vi "Clear Results.vi"(8 "error in (no error)":errorcluster, 11 "Results Manager in":refnum<class "Results Manager.lvclass">) -> (0 "error out":errorcluster, 3 "Results Manager out":refnum<class "Results Manager.lvclass">)   [LabVIEW 2021, in "Sequence Engine.lvlib" / "Results Manager.lvclass"]
uses:
  Results Manager.lvclass
  Test Result/Test Result.lvclass
  Results Manager.lvclass/Results Manager.ctl
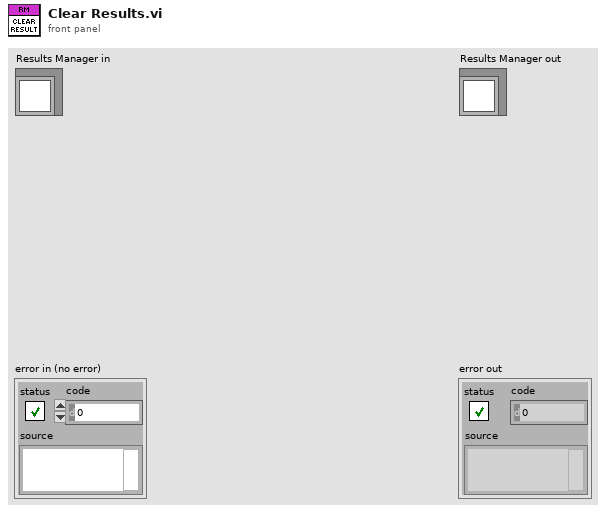
[diagram p1: front panel]
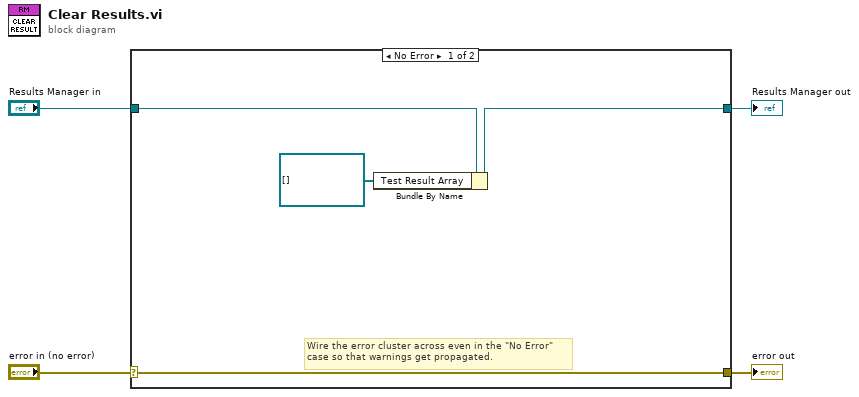
[diagram p0: block diagram]
diagram:
  n1 = case shown="No Error" "error in (no error)" {
    selector: "error in (no error)" -> [w7 w10]
    tunnel: [w7 w10] -> w3
    tunnel: [w6 w9] -> w1
    tunnel: "Results Manager in" -> [w8 w9]
    frame No Error {
      # "Wire the error cluster across even in the \"No Error\"\ncase so that warnings get propagated."
      n2 = Bundle By Name(cluster=w8, "Test Result Array"=refnum<class "Test Result.lvclass">[] []) -> (w6:refnum<class "Results Manager.lvclass">)
    }
    frame Error {
    }
  }
  "error out" <- w3
  "Results Manager out" <- w1
